vi "ActionOnError.vi"(8 "error in (no error)":errorcluster, 9 "Actual error":errorcluster, 11 "Channel Manager in":refnum<class "Channel Manager.lvclass">) -> (0 "error out":errorcluster, 3 "Channel Manager out":refnum<class "Channel Manager.lvclass">)   [LabVIEW 2024, in "Embedded TDMS Logger Engine.lvlib" / "Channel Manager.lvclass"]
uses:
  Channel Manager.lvclass
  Channel Manager.lvclass/Channel Manager.ctl
  Shared/File Classes/File/File.lvclass
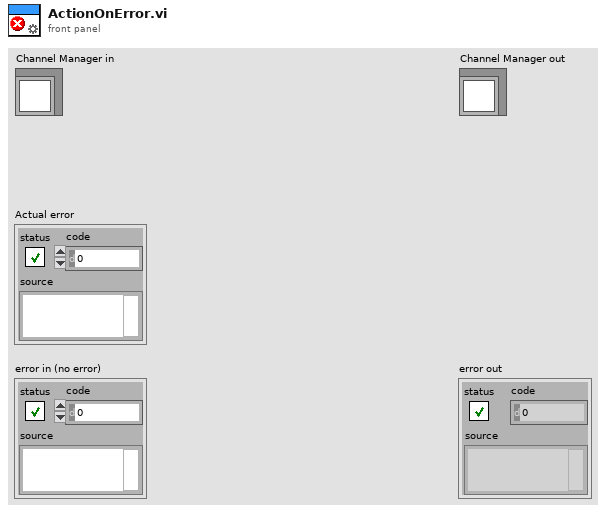
[diagram p1: front panel]
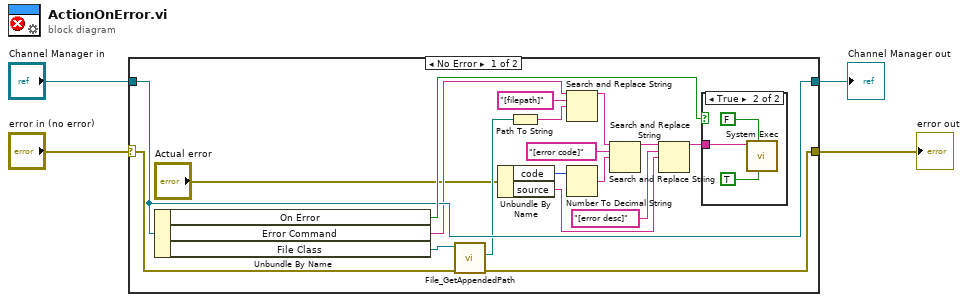
[diagram p0: block diagram]
diagram:
  n1 = case shown="No Error" "error in (no error)" {
    selector: "error in (no error)" -> [w19 w27]
    tunnel: [w16 w27] -> w3
    tunnel: [w21 w26] -> w1
    tunnel: "Channel Manager in" -> [w21 w26]
    frame No Error {
      n2 = Unbundle By Name(w21) -> ("On Error"=w22:bool, "Error Command"=w15:string, "File Class"=w20:refnum<class "File.lvclass">)
      n3 = call-dynamic "File_GetAppendedPath.vi"("error in (no error)"=w19, "File in"=w20) -> ("error out"=w16:errorcluster, "appended path"=w18:path)  [unwired: 7 in, 1 out]
      n4 = Unbundle By Name("Actual error") -> ("code"=w7:i32, "source"=w5:string)
      n5 = Path To String(path=w18) -> (string=w17:string)
      n6 = Search and Replace String(input string=w15, search string="[filepath]", replace string=w17) -> (result string=w13:string)  [unwired: 5 in, 3 out]
      n7 = Number To Decimal String(number=w7) -> (decimal integer string=w6:string)  [unwired: 1 in]
      n8 = Search and Replace String(input string=w13, search string="[error code]", replace string=w6) -> (result string=w12:string)  [unwired: 5 in, 3 out]
      n9 = Search and Replace String(input string=w12, search string="[error desc]", replace string=w5) -> (result string=w11:string)  [unwired: 5 in, 3 out]
      n10 = case shown="True" w22 {
        tunnel: w11 -> [_ w23]
        frame False {
        }
        frame True {
          n11 = call <vilib>:"System Exec.vi"("run minimized? (F)"=TRUE, "wait until completion? (T)"=FALSE, "command line"=w23) -> ()  [unwired: 5 in, 4 out]
        }
      }
    }
    frame Error {
    }
  }
  "error out" <- w3
  "Channel Manager out" <- w1
